vi "CCL.vi"(0 "System no.":i32=1 min=1 max=4 step=1, 2 "Command level":i32, 3 "Password":string, 5 "error in":errorcluster) -> (14 "Controller error":bool, 19 "error out":errorcluster)   [LabVIEW 2020]
doc: "If password is correct, this VI sets the command level of the controller and queries ERR?. Controller error is TRUE if selected system report error code not equal to zero. Use HLP?.vi to determine which commands are available in the current command level.\n\nC-413, C-867, C-877, C-884, C-891, E-517, E-518, E-709, E-710, E-712, E-725, E-727, E-753, E-754, E-755, E-870, E-871, E-872, E-873, E-874, F-206, M-8X0, Mercury_GCS: Command level can be 0 (only commands needed for normal operation are available) or 1 (all commands from command level 0 plus special commands for advanced users are available). Password for CCL 1 is \"ADVANCED\".\n\nC-867, C-884, Mercury_GCS: \n\nC-887, F-206, M-8X0: Only for GCS syntax version = GCS 2.0 or higher (check with CSV?.vi. If CSV?.vi is not supported, syntax version is GCS 1.0)."
panel:
  # "If password is correct, this vi sets the command level of the controller and \nqueries ERR?. See VI description for available levels. Use \"HLP?.vi\" to determine\nwhich commands are available in the current command level."
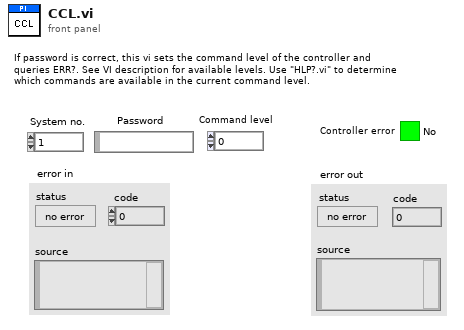
[diagram p1: front panel]
types:
  T1 = enum16{"Disable error check", "Force error check", "Use global settings"}
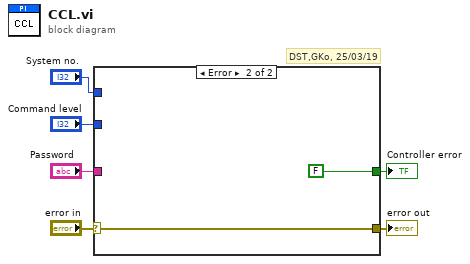
[diagram p0: block diagram]
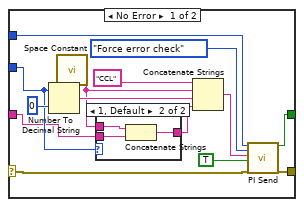
[diagram p2: hidden frame]
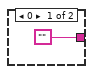
[diagram p3: hidden frame]
diagram:
  # "DST,GKo, 25/03/19"
  n1 = case shown="Error" "error in" {
    selector: "error in" -> [w11 w25]
    tunnel: [w15 w25] -> w6
    tunnel: "System no." -> [w19 _]
    tunnel: "Password" -> [w8 _]
    tunnel: [w14 FALSE ("Controller error")] -> w3
    tunnel: "Command level" -> [w10 _]
    frame No Error {
      n2 = Number To Decimal String(number=w10, width (-)=i16 0) -> (decimal integer string=w16:string)
      n3 = call "Space Constant.vi"() -> ("String"=w7:string)
      n4 = case shown="1, Default" w10 {
        tunnel: ["" w22] -> w9
        tunnel: w8 -> [_ w23]
        tunnel: w7 -> [_ w24]
        frame 0 {
        }
        frame 1, Default {
          n5 = Concatenate Strings(w24, w23) -> (w22:string)
        }
      }
      n6 = Concatenate Strings("CCL", w7, w16, w9) -> (w18:string)
      n7 = call "PI Send.vi"("System no."=w19, "Error check settings"=T1."Force error check", "String to send"=w18, "Attach termination char.?"=TRUE ("Attach Linefeed?"), "error in"=w11) -> ("Controller error"=w14:bool, "error out"=w15:errorcluster)  [unwired: 1 in, 12 out]
    }
    frame Error {
    }
  }
  "error out" <- w6
  "Controller error" <- w3
